vi "Flow Settings Dialog.vi"(8 "error in (no error)":errorcluster, 11 "Flow Module Config In":T1={"GUID"="", "Drop Coords"={"Horizontal"=0, "Vertical"=0}, "Process Name"="", "User name"="", "Queue Name"="", "Settings"={"Cycle Period"=500.0, "Flow Meter Type"="", "Bronkhorst M13 Settings"={"VISA resource name"="", "Simulated?"=FALSE, "Smoothing Steps"=1}, "Bronkhorst M14 Settings"={"VISA resource name"="", "Simulated?"=FALSE, "Smoothing Steps"=1}, "Reset Totalizer"=FALSE}, "Load Count"=0} {"Settings"."Bronkhorst M14 Settings"."Smoothing Steps" min=1 step=1; "Settings"."Bronkhorst M13 Settings"."Smoothing Steps" min=1 step=1}) -> (0 "error out":errorcluster, 1 "Cancelled?":bool=TRUE, 2 "UI Refresh Needed?":bool, 3 "Flow Module Config Out":T1={"GUID"="", "Drop Coords"={"Horizontal"=0, "Vertical"=0}, "Process Name"="", "User name"="", "Queue Name"="", "Settings"={"Cycle Period"=500.0, "Flow Meter Type"="", "Bronkhorst M13 Settings"={"VISA resource name"="", "Simulated?"=FALSE, "Smoothing Steps"=1}, "Bronkhorst M14 Settings"={"VISA resource name"="", "Simulated?"=FALSE, "Smoothing Steps"=1}, "Reset Totalizer"=FALSE}, "Load Count"=0} {"Settings"."Bronkhorst M14 Settings"."Smoothing Steps" min=1 step=1; "Settings"."Bronkhorst M13 Settings"."Smoothing Steps" min=1 step=1})   [LabVIEW 2018, in "Flow Module.lvlib"]
doc: "Dialog for selecting user specified settings."
uses:
  Flow Module.lvlib
  Feed Module/Controls/Flow Module Settings Cluster.ctl
  Bronkhorst M13 Flow Meter/Settings Cluster.ctl
  Bronkhorst M14 Flow Meter/Settings Cluster.ctl
  Feed Module/Controls/Flow Module Config Cluster.ctl
  <vilib>/Utility/miscctls.llb/LVPoint32TypeDef.ctl
  <vilib>/Utility/xml.llb/Write to XML File(string).vi
  Settings/Settings.lvlib
  Bronkhorst M13 Flow Meter/Bronkhorst M13 Flow Meter.lvlib
  Bronkhorst M14 Flow Meter/Bronkhorst M14 Flow Meter.lvlib
panel:
  in  "Module Name":string
  in  "Flow Meter Configuration":T3={"Cycle Period"=500.0, "Flow Meter Type"="Default", "Bronkhorst M13 Settings"={"VISA resource name"="", "Simulated?"=FALSE, "Smoothing Steps"=1}, "Bronkhorst M14 Settings"={"VISA resource name"="", "Simulated?"=FALSE, "Smoothing Steps"=1}, "Reset Totalizer"=FALSE} {"Bronkhorst M14 Settings"."Smoothing Steps" min=1 step=1; "Bronkhorst M13 Settings"."Smoothing Steps" min=1 step=1}
  in  "Cancel Button":bool
  in  "OK Button":bool
  # "Non visible portion of dialog (needed for connector pane)."
  # "Flow Meter Settings"
  # "Flow Meter Settings"
  # "Flow Meter Settings"
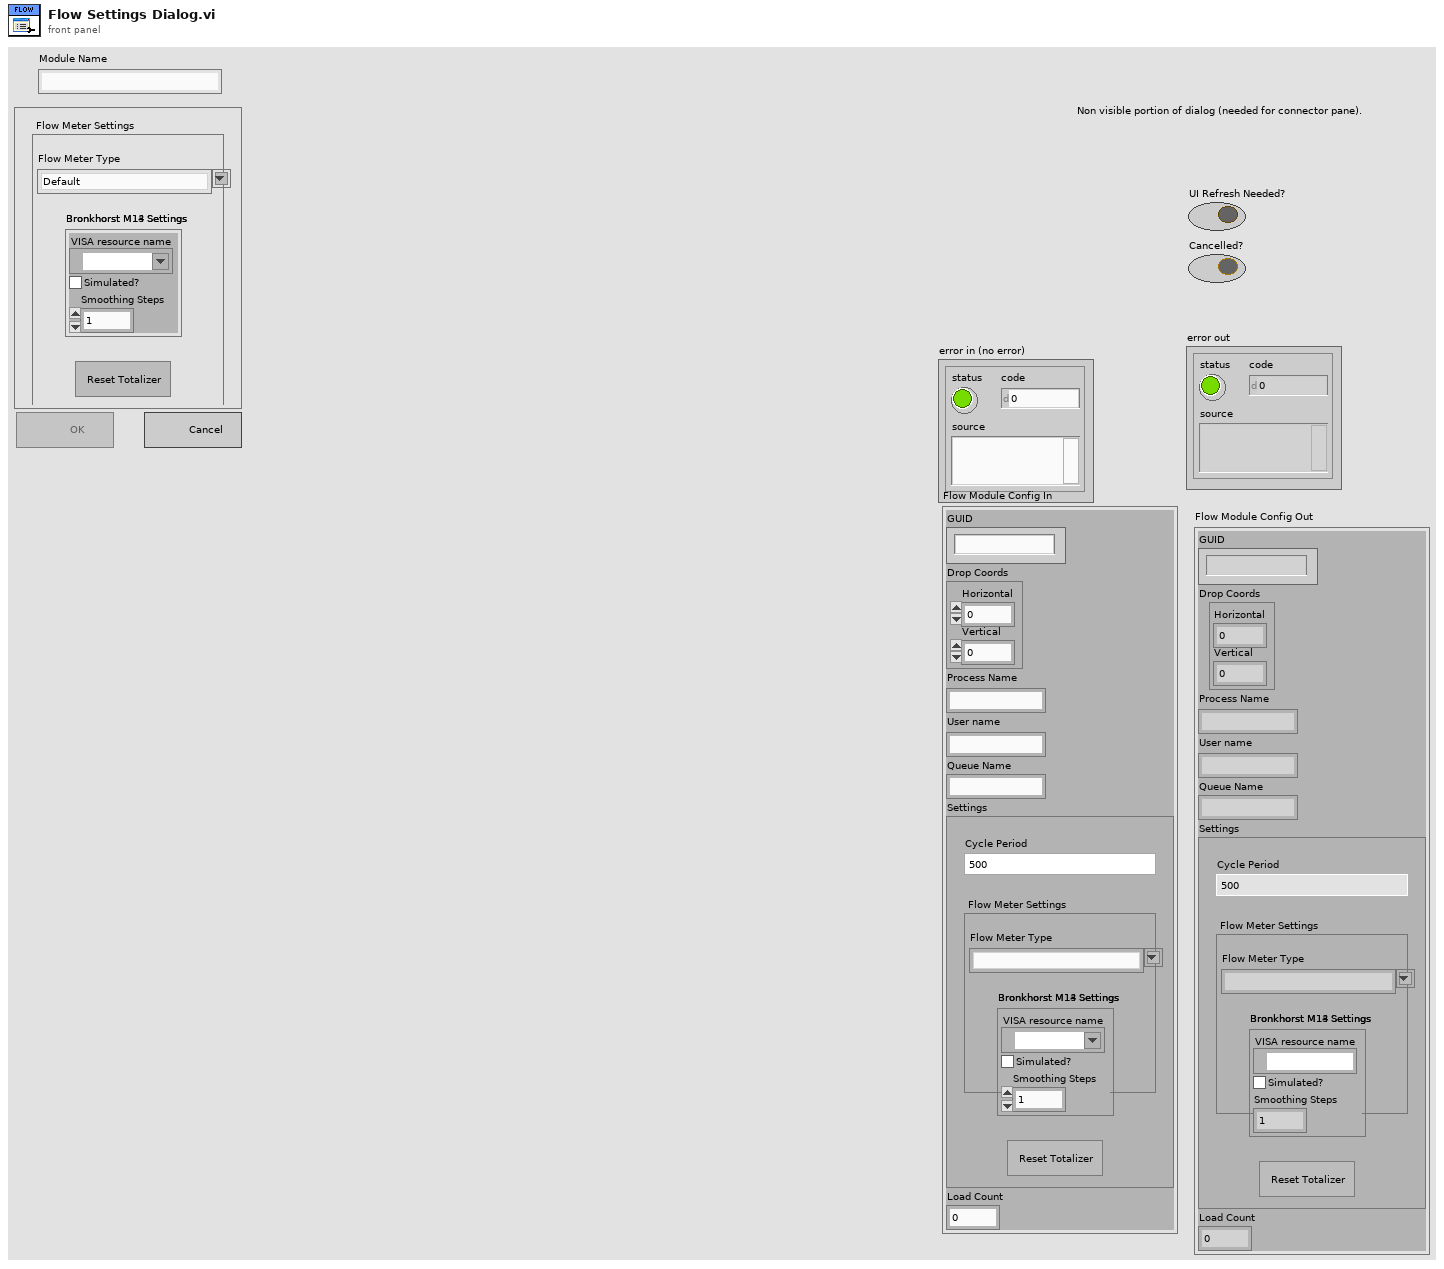
[diagram p1: front panel]
types:
  T1 = typedef "Flow Module.lvlib/Flow Module Config Cluster.ctl" = cluster{"GUID":string, "Drop Coords":T2, "Process Name":string, "User name":string, "Queue Name":string, "Settings":T3, "Load Count":i32}
  T2 = typedef "LVPoint32TypeDef.ctl" = cluster{"Horizontal":i32, "Vertical":i32}
  T3 = typedef "Flow Module.lvlib/Flow Module Settings Cluster.ctl" = cluster{"Cycle Period":dbl, "Flow Meter Type":string, "Bronkhorst M13 Settings":T4, "Bronkhorst M14 Settings":T5, "Reset Totalizer":bool}
  T4 = typedef "Bronkhorst M13 Flow Meter.lvlib/Settings Cluster.ctl" = cluster{"VISA resource name":refnum<visa-resource-name>, "Simulated?":bool, "Smoothing Steps":i32}
  T5 = typedef "Bronkhorst M14 Flow Meter.lvlib/Settings Cluster.ctl" = cluster{"VISA resource name":refnum<visa-resource-name>, "Simulated?":bool, "Smoothing Steps":i32}
  T6 = enum8{"Enabled", "Disabled", "Disabled and Grayed Out"}
  T7 = cluster{"Cycle Period":dbl, "Flow Meter Type":string, "Bronkhorst M13 Settings":T4, "Bronkhorst M14 Settings":T5, bool}
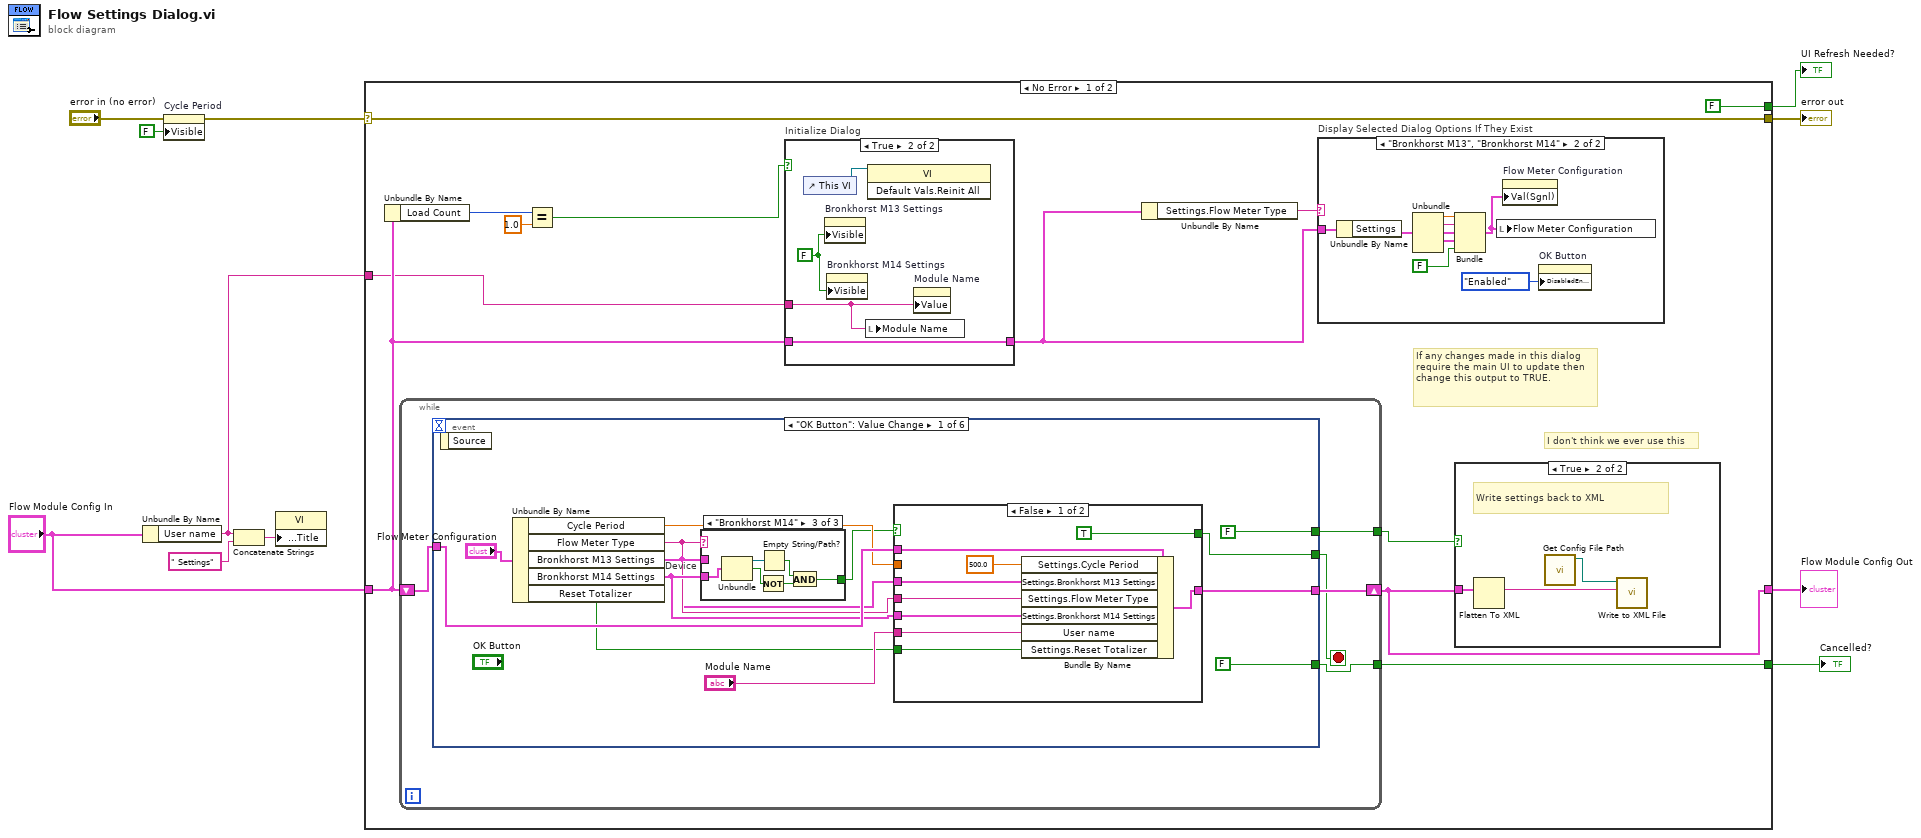
[diagram p0: block diagram]
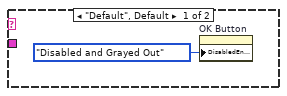
[diagram p2: hidden frame]
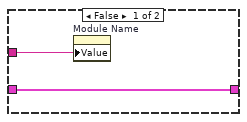
[diagram p3: hidden frame]
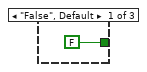
[diagram p4: hidden frame]
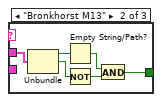
[diagram p5: hidden frame]
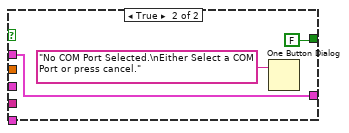
[diagram p6: hidden frame]
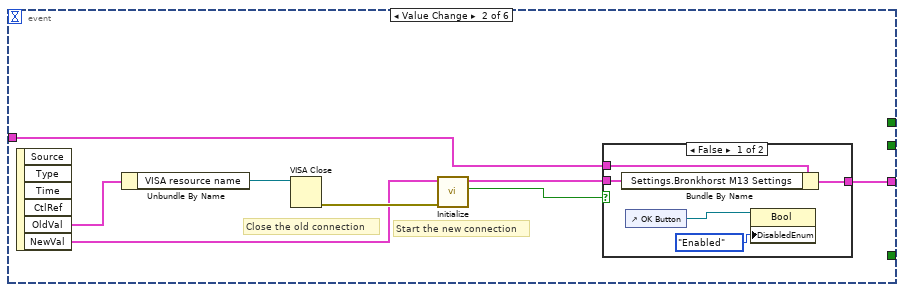
[diagram p7: hidden frame]
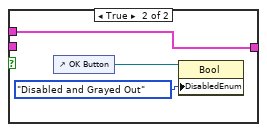
[diagram p8: hidden frame]
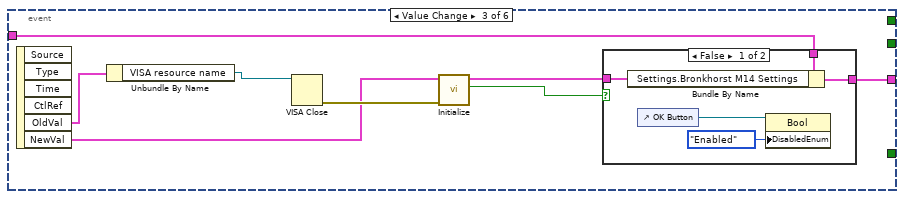
[diagram p9: hidden frame]
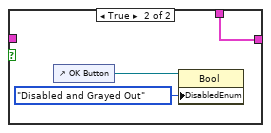
[diagram p10: hidden frame]
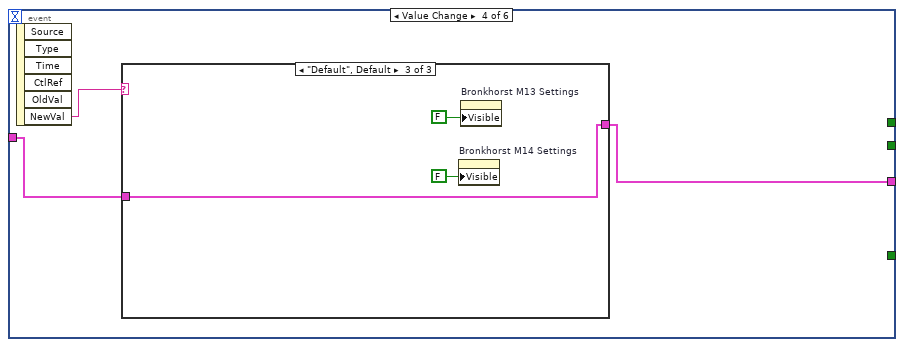
[diagram p11: hidden frame]
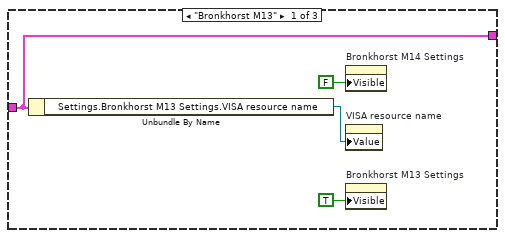
[diagram p12: hidden frame]
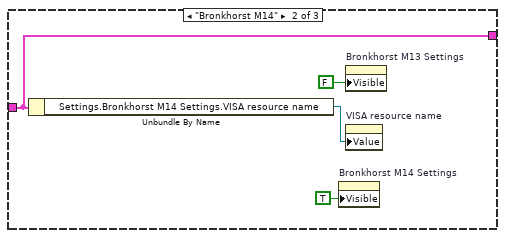
[diagram p13: hidden frame]
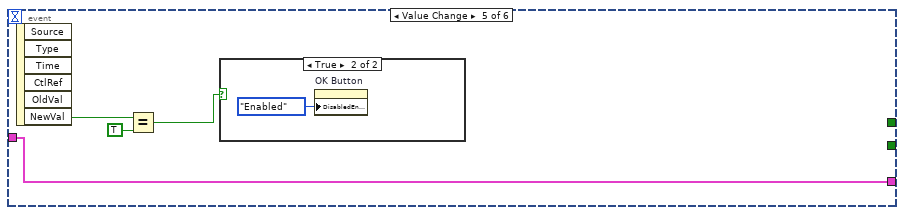
[diagram p14: hidden frame]
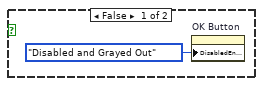
[diagram p15: hidden frame]
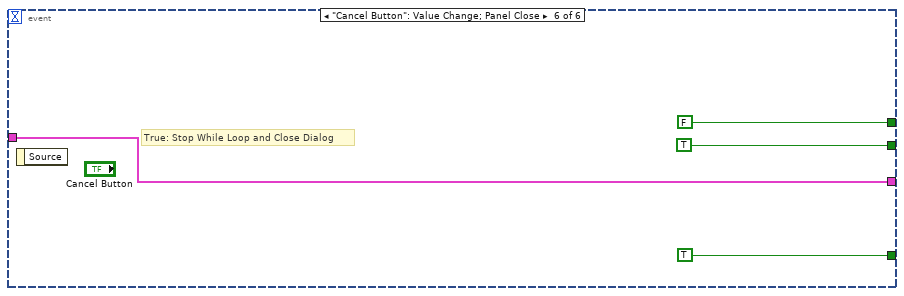
[diagram p16: hidden frame]
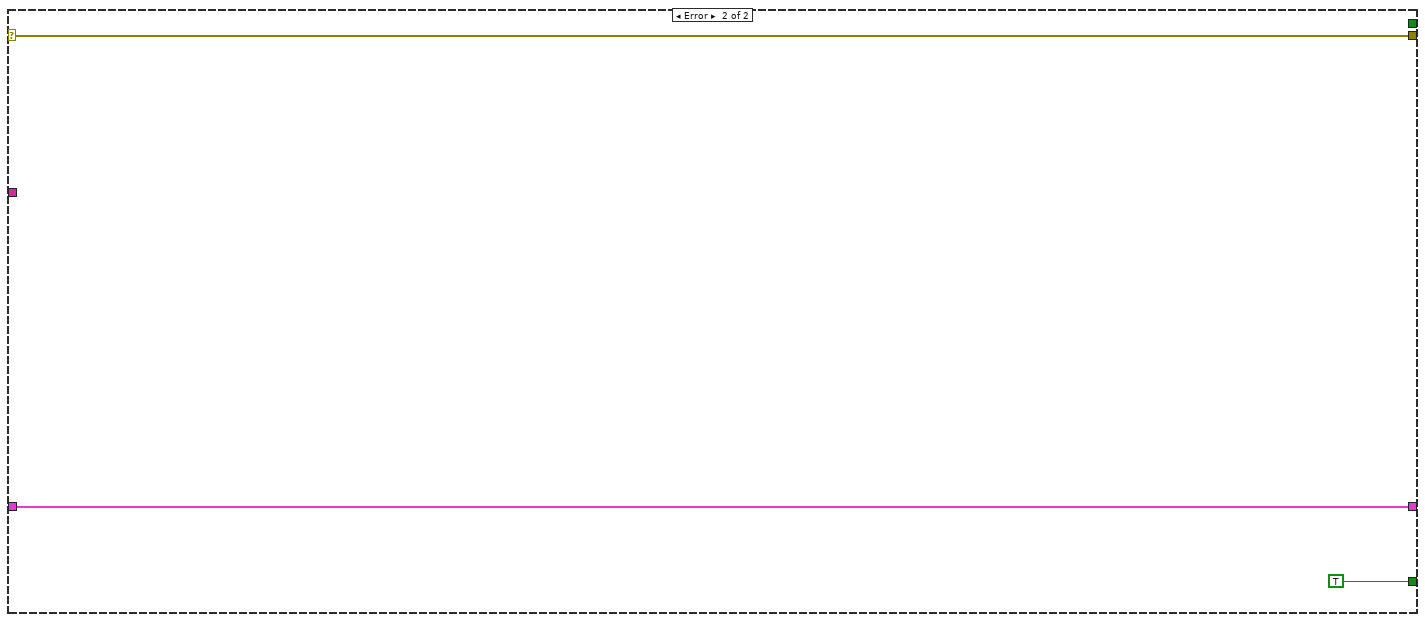
[diagram p18: hidden frame]
diagram:
  n1 = Unbundle By Name("Flow Module Config In") -> ("User name"=w1:string)
  n2 = property on="Cycle Period" class="DigNum (strict)"(error in="error in (no error)", "Visible"=FALSE) -> (error out=w5:errorcluster)  [unwired: 1 in, 1 out]
  n3 = Concatenate Strings(w1, " Settings" ("string")) -> (w4:string)
  n4 = property class="VI"("Front Panel.Title"=w4) -> ()  [unwired: 2 in, 2 out]
  n5 = case shown="No Error" w5 {
    selector: w5 -> [w23 w144]
    tunnel: [w23 w144] -> w11
    tunnel: "Flow Module Config In" -> [w13 w143]
    tunnel: [w21 w143] -> w8
    tunnel: [FALSE ("UI Refresh Needed?") _] -> w10
    tunnel: [w17 TRUE ("UI Refresh Needed?")] -> w9
    tunnel: w1 -> [w12 _]
    frame No Error {
      # "I don't think we ever use this"
      # "If any changes made in this dialog require the main UI to update then change this output to TRUE."
      n6 = Unbundle By Name(w13) -> ("Load Count"=w20:i32)
      n7 = while {
        tunnel: [w44] -> w18
        tunnel: [w41] -> w17
        shift-right: [w43] -> w21
        shift-left: w13 -> [w40]
        stop <- w42 stop-if-true
        n8 = event shown="[0] \"OK Button\": Value Change" {
          selector: _ -> [_ _ _ _ _ _]
          dyn-events: _ -> [_ _ _ _ _ _]
          timeout: _ -> [_ _ _ _ _ _]
          tunnel: [w55 w89 w105 w116 w132 w138] -> w43
          tunnel: w40 -> [w54 w90 w106 w115 w132 w138]
          tunnel: [FALSE ("UI Refresh Needed?") _ _ _ _ FALSE ("UI Refresh Needed?")] -> w44
          tunnel: [w56 _ _ _ _ TRUE] -> w42
          tunnel: [FALSE ("UI Refresh Needed?") _ _ _ _ TRUE ("UI Refresh Needed?")] -> w41
          event "OK Button": Value Change {
            n9 = event-data() -> ()  [unwired: 1 in, 1 out]
            n10 = Unbundle By Name("Flow Meter Configuration") -> ("Cycle Period"=w52:dbl, "Flow Meter Type"=w47:string, "Bronkhorst M13 Settings"=w46:T4, "Bronkhorst M14 Settings"=w49:T5, "Reset Totalizer"=w45:bool)
            n11 = case "Device" shown="\"Bronkhorst M14\"" w47 {
              tunnel: [FALSE w60 w66] -> w50
              tunnel: w49 -> [_ _ w65]
              tunnel: w46 -> [_ w59 _]
              frame "False", Default {
              }
              frame "Bronkhorst M13" {
                n12 = Unbundle(w59) -> ("VISA resource name"=w64:refnum<visa-resource-name>, "Simulated?"=w63:bool)  [unwired: 1 out]
                n13 = Empty String/Path?(string/path=w64) -> (empty?=w61:bool)
                n14 = Not(x=w63) -> (.not. x?=w62:bool)
                n15 = And(x=w61, y=w62) -> (x .and. y?=w60:bool)
              }
              frame "Bronkhorst M14" {
                n16 = Unbundle(w65) -> ("VISA resource name"=w70:refnum<visa-resource-name>, "Simulated?"=w69:bool)  [unwired: 1 out]
                n17 = Not(x=w69) -> (.not. x?=w68:bool)
                n18 = Empty String/Path?(string/path=w70) -> (empty?=w67:bool)
                n19 = And(x=w67, y=w68) -> (x .and. y?=w66:bool)
              }
            }
            n20 = case shown="False" w50 {
              tunnel: [TRUE FALSE] -> w56
              tunnel: [w78 w81] -> w55
              tunnel: w54 -> [w77 w81]
              tunnel: w47 -> [w76 _]
              tunnel: w46 -> [w75 _]
              tunnel: w52 -> [_ _]
              tunnel: w49 -> [w74 _]
              tunnel: "Module Name" -> [w72 _]
              tunnel: w45 -> [w71 _]
              frame False {
                n21 = Bundle By Name(cluster=w77, "Settings.Cycle Period"=500.0, "Settings.Bronkhorst M13 Settings"=w75, "Settings.Flow Meter Type"=w76, "Settings.Bronkhorst M14 Settings"=w74, "User name"=w72, "Settings.Reset Totalizer"=w71) -> (w78:T1)
              }
              frame True {
                n22 = One Button Dialog(message="No COM Port Selected.\nEither Select a COM Port or press cancel.") -> ()  [unwired: 1 in, 1 out]
              }
            }
          }
          event Value Change {
            # "Start the new connection"
            # "Close the old connection"
            n23 = event-data() -> ("OldVal"=w85:T4, "NewVal"=w83:T4)  [unwired: 1 in, 4 out]
            n24 = Unbundle By Name(w85) -> ("VISA resource name"=w84:refnum<visa-resource-name>)
            n25 = VISA Close(VISA resource name=w84) -> (error out=w87:errorcluster)  [unwired: 1 in]
            n26 = call "Initialize.vi"("error in (no error)"=w87, "Bronkhorst Settings in"=w83) -> ("No Meter Connnected"=w86:bool, "Bronkhorst Settings out"=w88:T4)  [unwired: 7 in, 1 out]
            n27 = case shown="False" w86 {
              tunnel: w90 -> [w95 w98]
              tunnel: [w94 w98] -> w89
              tunnel: w88 -> [w93 _]
              frame False {
                n28 = Bundle By Name(cluster=w95, "Settings.Bronkhorst M13 Settings"=w93) -> (w94:T1)
                n29 = control-ref of="OK Button"() -> (w91:refnum<vi>)
                n30 = property class="Bool"(reference=w91, "DisabledEnum"=T6."Enabled" ("Disabled")) -> ()  [unwired: 1 in, 2 out]
              }
              frame True {
                n31 = control-ref of="OK Button"() -> (w96:refnum<vi>)
                n32 = property class="Bool"(reference=w96, "DisabledEnum"=T6."Disabled and Grayed Out" ("Disabled")) -> ()  [unwired: 1 in, 2 out]
              }
            }
          }
          event Value Change {
            n33 = event-data() -> ("OldVal"=w101:T5, "NewVal"=w99:T5)  [unwired: 1 in, 4 out]
            n34 = Unbundle By Name(w101) -> ("VISA resource name"=w100:refnum<visa-resource-name>)
            n35 = VISA Close(VISA resource name=w100) -> (error out=w103:errorcluster)  [unwired: 1 in]
            n36 = call "Initialize.vi"("error in (no error)"=w103, "Bronkhorst Settings in"=w99) -> ("No Meter Connected"=w102:bool, "Bronkhorst Settings out"=w104:T5)  [unwired: 7 in, 1 out]
            n37 = case shown="False" w102 {
              tunnel: w106 -> [w111 w114]
              tunnel: [w110 w114] -> w105
              tunnel: w104 -> [w109 _]
              frame False {
                n38 = Bundle By Name(cluster=w111, "Settings.Bronkhorst M14 Settings"=w109) -> (w110:T1)
                n39 = control-ref of="OK Button"() -> (w108:refnum<vi>)
                n40 = property class="Bool"(reference=w108, "DisabledEnum"=T6."Enabled" ("Disabled")) -> ()  [unwired: 1 in, 2 out]
              }
              frame True {
                n41 = control-ref of="OK Button"() -> (w113:refnum<vi>)
                n42 = property class="Bool"(reference=w113, "DisabledEnum"=T6."Disabled and Grayed Out" ("Disabled")) -> ()  [unwired: 1 in, 2 out]
              }
            }
          }
          event Value Change {
            n43 = event-data() -> ("NewVal"=w117:string)  [unwired: 1 in, 5 out]
            n44 = case shown="\"Default\", Default" w117 {
              tunnel: [w119 w123 w128] -> w116
              tunnel: w115 -> [w119 w123 w128]
              frame "Bronkhorst M13" {
                n45 = Unbundle By Name(w119) -> ("Settings.Bronkhorst M13 Settings.VISA resource name"=w121:refnum<visa-resource-name>)
                n46 = property on="Bronkhorst M14 Settings" class="Clust (strict)"("Visible"=FALSE) -> ()  [unwired: 2 in, 2 out]
                n47 = property on="VISA resource name" class="VISAName"("Value"=w121) -> ()  [unwired: 2 in, 2 out]
                n48 = property on="Bronkhorst M13 Settings" class="Clust (strict)"("Visible"=TRUE) -> ()  [unwired: 2 in, 2 out]
              }
              frame "Bronkhorst M14" {
                n49 = Unbundle By Name(w123) -> ("Settings.Bronkhorst M14 Settings.VISA resource name"=w125:refnum<visa-resource-name>)
                n50 = property on="Bronkhorst M14 Settings" class="Clust (strict)"("Visible"=TRUE) -> ()  [unwired: 2 in, 2 out]
                n51 = property on="Bronkhorst M13 Settings" class="Clust (strict)"("Visible"=FALSE) -> ()  [unwired: 2 in, 2 out]
                n52 = property on="VISA resource name" class="VISAName"("Value"=w125) -> ()  [unwired: 2 in, 2 out]
              }
              frame "Default", Default {
                n53 = property on="Bronkhorst M14 Settings" class="Clust (strict)"("Visible"=FALSE) -> ()  [unwired: 2 in, 2 out]
                n54 = property on="Bronkhorst M13 Settings" class="Clust (strict)"("Visible"=FALSE) -> ()  [unwired: 2 in, 2 out]
              }
            }
          }
          event Value Change {
            n55 = event-data() -> ("NewVal"=w130:bool)  [unwired: 1 in, 5 out]
            n56 = Equal?(x=w130, y=TRUE) -> (x = y?=w129:bool)
            n57 = case shown="True" w129 {
              frame False {
                n58 = property on="OK Button" class="Bool"("DisabledEnum"=T6."Disabled and Grayed Out" ("Disabled")) -> ()  [unwired: 2 in, 2 out]
              }
              frame True {
                n59 = property on="OK Button" class="Bool"("DisabledEnum"=T6."Enabled" ("Disabled")) -> ()  [unwired: 2 in, 2 out]
              }
            }
          }
          event "Cancel Button": Value Change; Panel Close {
            # "True: Stop While Loop and Close Dialog"
            n60 = event-data() -> ()  [unwired: 1 in, 1 out]
          }
        }
      }
      n61 = Equal?(x=w20, y=1.0) -> (x = y?=w16:bool)
      n62 = case "Initialize Dialog" shown="True" w16 {
        tunnel: w13 -> [w35 w38]
        tunnel: [w35 w38] -> w14
        tunnel: w12 -> [w34 w37]
        frame False {
          n63 = property on="Module Name" class="Str"("Value"=w34) -> ()  [unwired: 2 in, 2 out]
        }
        frame True {
          w36 = FALSE ("Visible")
          n64 = control-ref of="This VI"() -> (w39:refnum<vi>)
          n65 = property on="Bronkhorst M13 Settings" class="Clust (strict)"("Visible"=w36) -> ()  [unwired: 2 in, 2 out]
          n66 = property on="Bronkhorst M14 Settings" class="Clust (strict)"("Visible"=w36) -> ()  [unwired: 2 in, 2 out]
          n67 = local write "Module Name"(w37) -> ()
          n68 = invoke class="VI" method="Default Vals.Reinit All"(reference=w39) -> ()  [unwired: 2 in, 3 out]
          n69 = property on="Module Name" class="Str"("Value"=w37) -> ()  [unwired: 2 in, 2 out]
        }
      }
      n70 = Unbundle By Name(w14) -> ("Settings.Flow Meter Type"=w15:string)
      n71 = case "Display Selected Dialog Options If They Exist" shown="\"Bronkhorst M13\", \"Bronkhorst M14\"" w15 {
        tunnel: w14 -> [_ w30]
        frame "Default", Default {
          n72 = property on="OK Button" class="Bool"("DisabledEnum"=T6."Disabled and Grayed Out" ("Disabled")) -> ()  [unwired: 2 in, 2 out]
        }
        frame "Bronkhorst M13", "Bronkhorst M14" {
          n73 = Unbundle By Name(w30) -> ("Settings"=w27:T3)
          n74 = Unbundle(w27) -> ("Cycle Period"=w32:dbl, "Flow Meter Type"=w33:string, "Bronkhorst M13 Settings"=w31:T4, "Bronkhorst M14 Settings"=w29:T5)  [unwired: 1 out]
          n75 = Bundle("Cycle Period"=w32, "Flow Meter Type"=w33, "Bronkhorst M13 Settings"=w31, "Bronkhorst M14 Settings"=w29, FALSE) -> (w26:T7)  [unwired: 1 in]
          n76 = local write "Flow Meter Configuration"(w26) -> ()
          n77 = property on="Flow Meter Configuration" class="Clust (strict)"("Val(Sgnl)"=w26) -> ()  [unwired: 2 in, 2 out]
          n78 = property on="OK Button" class="Bool"("DisabledEnum"=T6."Enabled" ("Disabled")) -> ()  [unwired: 2 in, 2 out]
        }
      }
      n79 = case shown="True" w18 {
        tunnel: w21 -> [_ w140]
        frame False {
        }
        frame True {
          # "Write settings back to XML"
          n80 = Flatten To XML(anything=w140) -> (xml string=w139:string)
          n81 = call "Get Config File Path.vi"() -> ("XML File Path"=w141:path)  [unwired: 10 in, 1 out]
          n82 = call-poly <vilib>:"Write to XML File.vi"("XML Input"=w139, "XML File Path"=w141) -> ()  [unwired: 7 in, 3 out]
        }
      }
    }
    frame Error {
    }
  }
  "UI Refresh Needed?" <- w10
  "error out" <- w11
  "Cancelled?" <- w9
  "Flow Module Config Out" <- w8
